vi "DataLog Dump Tag Buffer.vi"(9 "tag index":i32=-1, 11 "error in (no error)":errorcluster) -> (6 "read index":i32, 8 "points":T1[](array[typedef]) {"value" format="%.3e"; "time" format="%<%H:%M:%S%2u\n%Y/%m/%d>T"}, 10 "tag index dup":i32, 15 "error out":errorcluster)   [LabVIEW 2012]
doc: "Dumps as much of the content of the buffer of a tag as possible. The content is returned as an array of points."
uses:
  typedefs/clusters/t_DataLog Point.ctl
  typedefs/t_DataLog Tag Buffers Methods.ctl
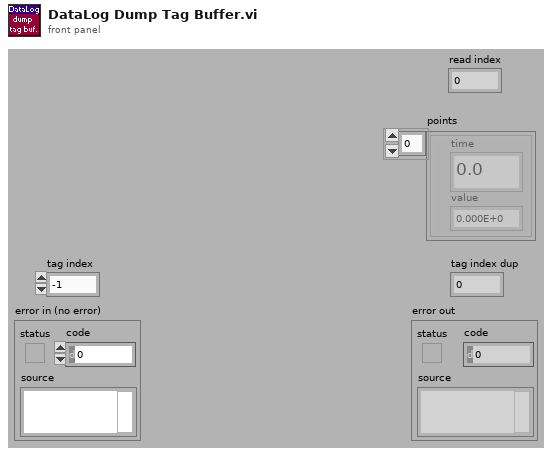
[diagram p1: front panel]
types:
  T1 = typedef "t_DataLog Point.ctl" = cluster{"time":dbl, "value":dbl}
  T2 = typedef "t_DataLog Tag Buffers Methods.ctl" = enum16{"initialize", "inert", "write", "read", "read oldest", "read last", "cleanup"}
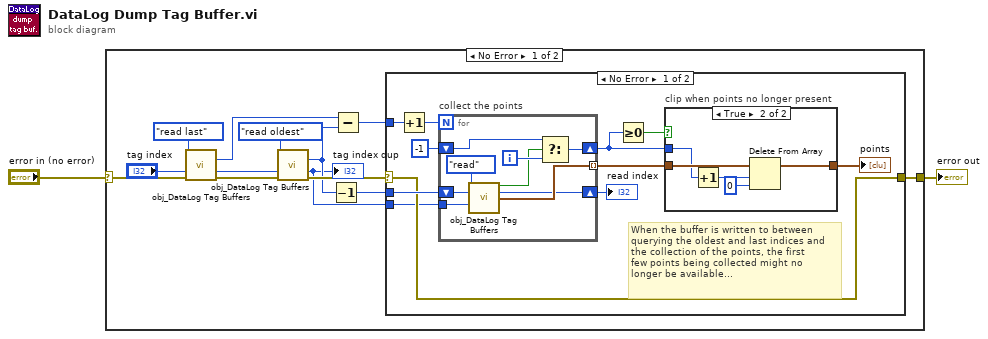
[diagram p0: block diagram]
diagram:
  n1 = case shown="No Error" "error in (no error)" {
    selector: "error in (no error)" -> [w9 w43]
    tunnel: [w8 w43] -> w1
    frame No Error {
      n2 = call "obj_DataLog Tag Buffers.vi"("method"=t_DataLog_Tag_Buffers_Methods."read last", "tag index"="tag index", "error in (no error)"=w9) -> ("read index out"=w7:i32, "tag index dup"=w4:i32, "error out"=w13:errorcluster)  [unwired: 8 in, 2 out]
      n3 = call "obj_DataLog Tag Buffers.vi"("method"=t_DataLog_Tag_Buffers_Methods."read oldest", "tag index"=w4, "error in (no error)"=w13) -> ("read index out"=w6:i32, "tag index dup"=w3:i32, "error out"=w12:errorcluster)  [unwired: 8 in, 2 out]
      "tag index dup" <- w3
      n4 = Decrement(x=w6) -> (x-1=w10:i32)
      n5 = Subtract(x=w7, y=w6) -> (x-y=w11:i32)
      n6 = case shown="No Error" w12 {
        selector: w12 -> [w18 w42]
        tunnel: w11 -> [w26 _]
        tunnel: w10 -> [w25 _]
        tunnel: [w18 w42] -> w8
        tunnel: w3 -> [w17 _]
        frame No Error {
          # "When the buffer is written to between\nquerying the oldest and last indices and\nthe collection of the points, the first\nfew points being collected might no\nlonger be available..."
          n7 = Increment(x=w26) -> (x+1=w16:i32)
          n8 = for "collect the points" {
            N: w16 -> [_]
            shift-right: [w34] -> w23
            shift-left: w25 -> [w35]
            tunnel: [w40] -> w20 mode=indexing
            shift-right: [w39] -> w21
            shift-left: -1 -> [w38]
            tunnel: w17 -> [w33]
            i -> [w37]
            n9 = call "obj_DataLog Tag Buffers.vi"("method"=t_DataLog_Tag_Buffers_Methods."read", "read index in"=w35, "tag index"=w33) -> ("available?"=w36:bool, "read index out"=w34:i32, "point out"=w40:T1)  [unwired: 8 in, 2 out]
            n10 = Select(t=w38, s=w36, f=w37) -> (s? t:f=w39:i32)
          }
          "read index" <- w23
          n11 = Greater Or Equal To 0?(x=w21) -> (x >= 0?=w22:bool)
          n12 = case "clip when points no longer present" shown="True" w22 {
            tunnel: w21 -> [_ w30]
            tunnel: w20 -> [w27 w32]
            tunnel: [w27 w28] -> w19
            frame False {
            }
            frame True {
              n13 = Increment(x=w30) -> (x+1=w29:i32)
              n14 = Delete From Array(array=w32, length=w29, index=0) -> (array with subset deleted=w28:T1[])  [unwired: 1 out]
            }
          }
          "points" <- w19
        }
        frame Error {
        }
      }
    }
    frame Error {
    }
  }
  "error out" <- w1
